vi "Feature_whole(SubVI)_TV.vi"(0 "Binary Image":T1) -> (4 "P":dbl, 5 "rgb Hull Image 2":T1(plugin-control), 6 "SA":dbl, 7 "bw Hull Image 2":T1(plugin-control), 8 "SFD":sgl, 9 "Hull area":dbl, 10 "SW":dbl, 12 "IFD":sgl, 13 "top":i32, 14 "最小外接矩面积":dbl, 15 "SH":dbl)   [LabVIEW 2015]
uses:
  <vilib>/vision/Image Controls.llb/IMAQ Image.ctl
  <vilib>/vision/NI_Vision_Development_Module.lvlib
  fractaldim.dll
  TotalContoursConvexHull.dll
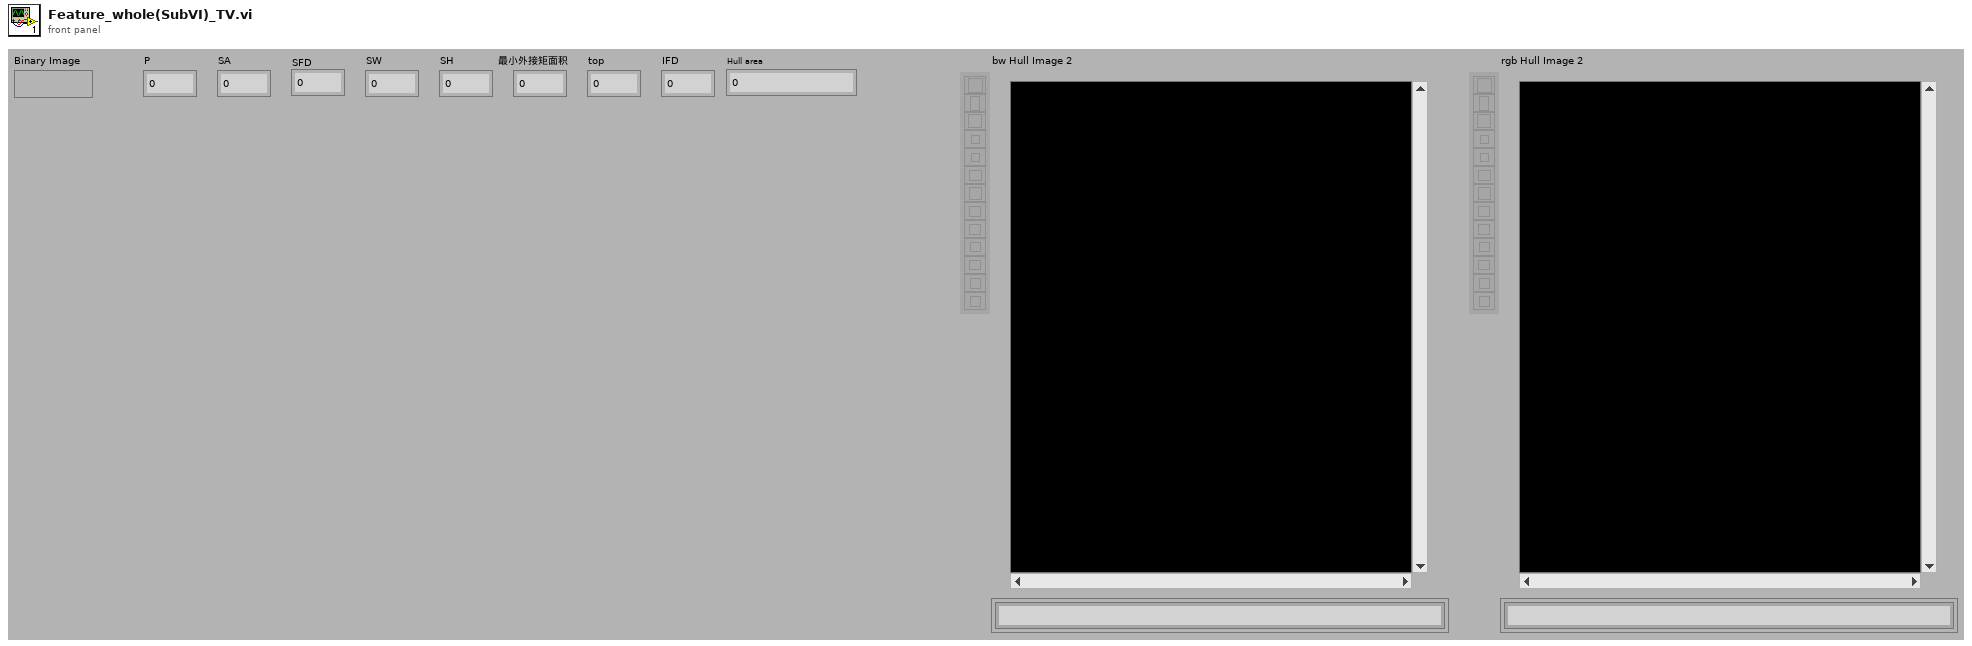
[diagram p1: front panel]
types:
  T1 = typedef "IMAQ Image.ctl" = refnum<image>
  T2 = typedef "Particle Parameters" = i32
  T3 = typedef "Image Type" = u32
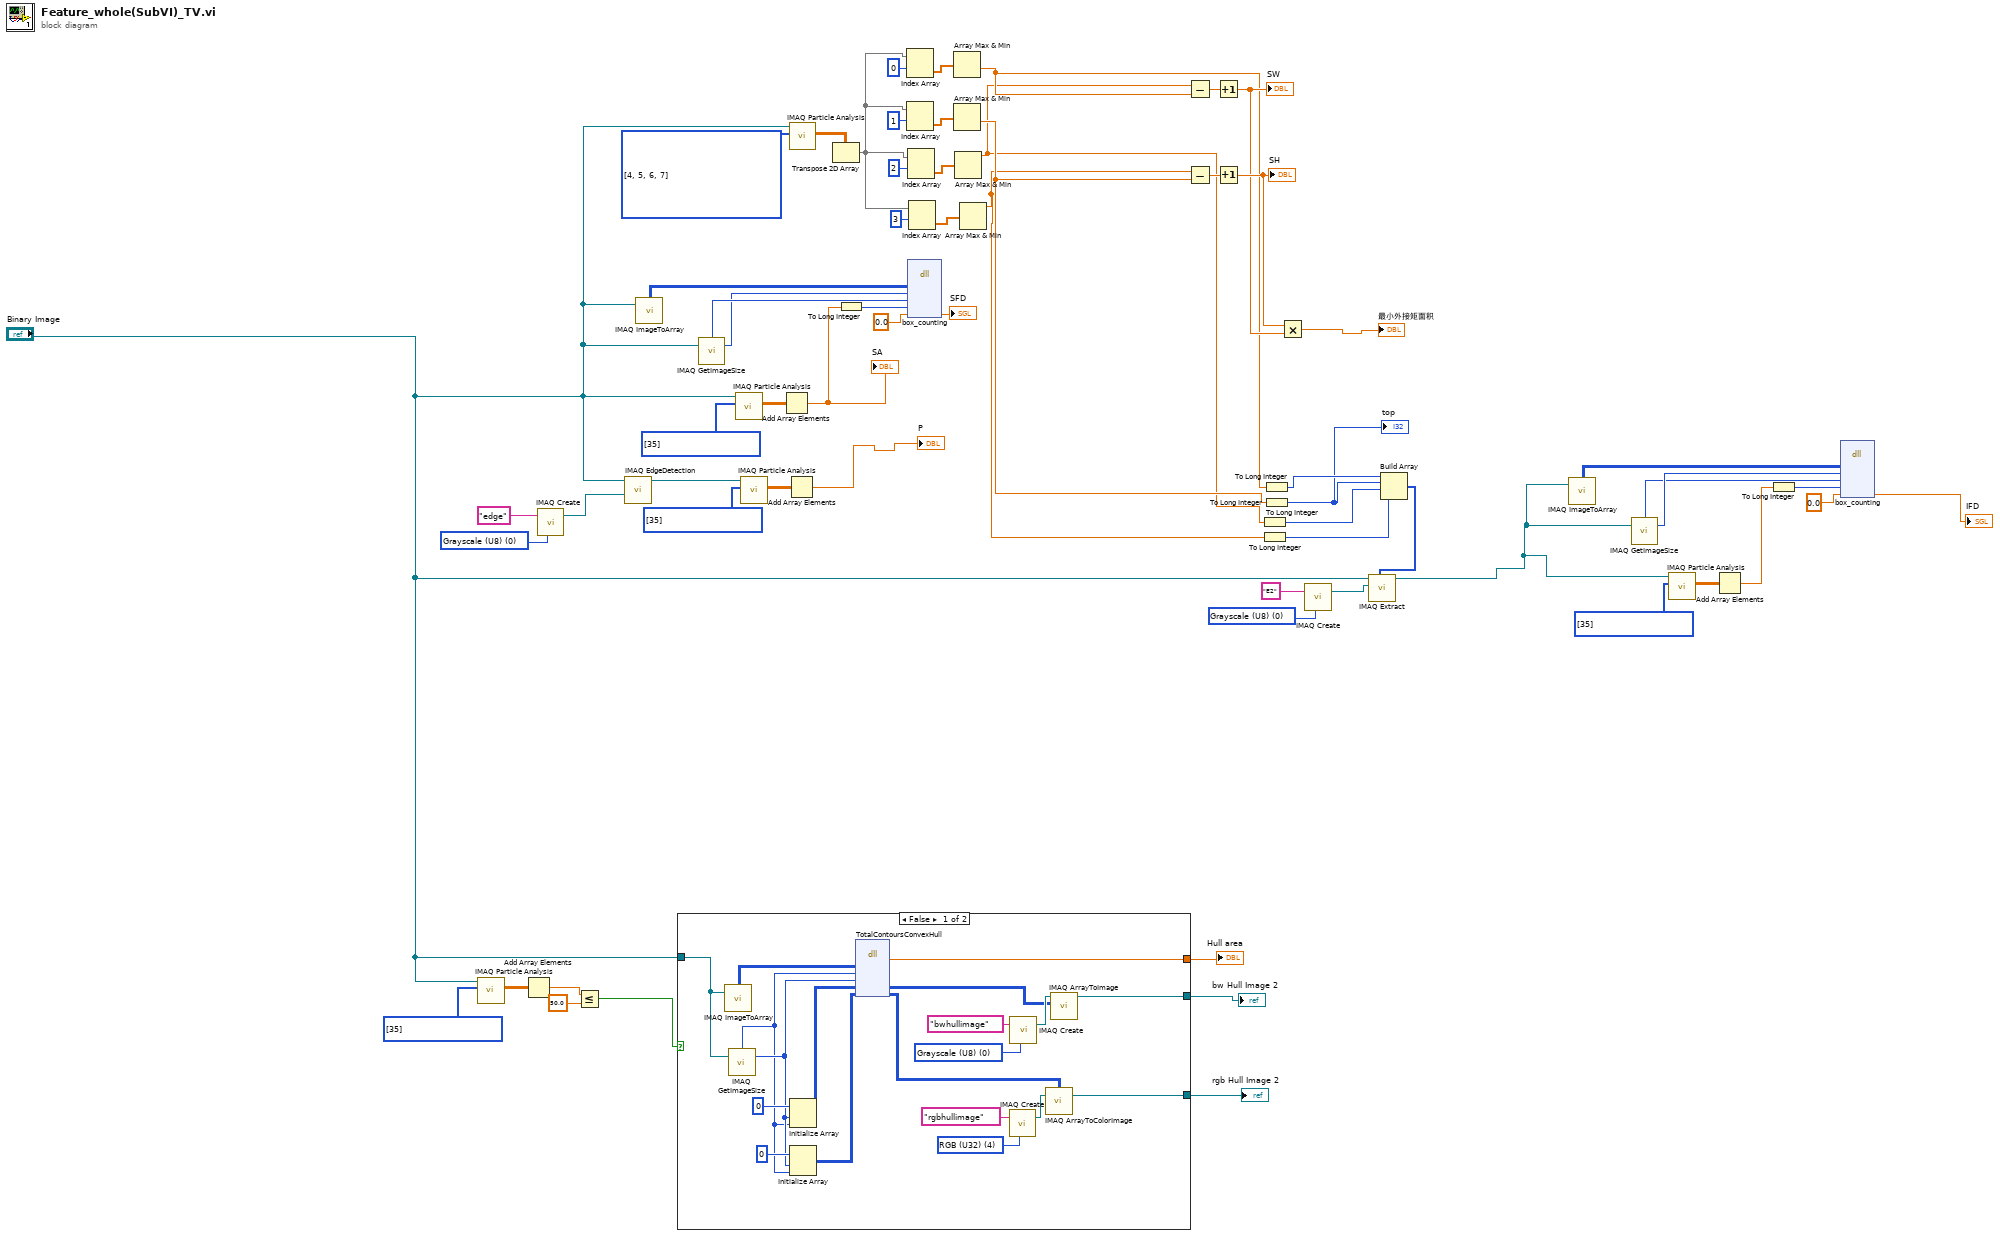
[diagram p0: block diagram]
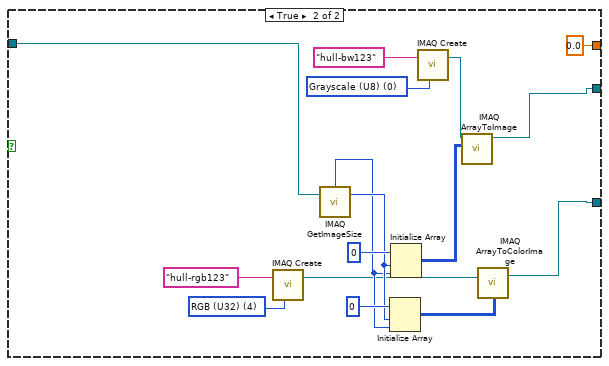
[diagram p2: hidden frame]
diagram:
  w7 = T2[] [35] items=["Center of Mass X", "Center of Mass Y", "First Pixel X", "First Pixel Y", "Bounding Rect Left", "Bounding Rect Top", "Bounding Rect Right", "Bounding Rect Bottom", "Max Feret Diameter Start X", "Max Feret Diameter Start Y", "Max Feret Diameter End X", "Max Feret Diameter End Y", "Max Horiz. Segment Length Left", "Max Horiz. Segment Length Right", "Max Horiz. Segment Length Row", "-", "Bounding Rect Width", "Bounding Rect Height", "Bounding Rect Diagonal", "Perimeter", "Convex Hull Perimeter", "Holes' Perimeter", "Max Feret Diameter", "Equivalent Ellipse Major Axis", "Equivalent Ellipse Minor Axis", "Equivalent Ellipse Minor Axis (Feret)", "Equivalent Rect Long Side", "Equivalent Rect Short Side", "Equivalent Rect Diagonal", "Equivalent Rect Short Side (Feret)", "Average Horiz. Segment Length", "Average Vert. Segment Length", "Hydraulic Radius", "Waddel Disk Diameter", "-", "Area", "Holes' Area", "Particle & Holes' Area", "Convex Hull Area", "Image Area", "-", "Number of Holes", "Number of Horiz. Segments", "Number of Vert. Segments", "-", "Orientation", "Max Feret Diameter Orientation", "-", "% Area/Image Area", "% Area/(Particle & Holes' Area)", "Ratio of Equivalent Ellipse Axes", "Ratio of Equivalent Rect Sides", "-", "Elongation Factor", "Compactness Factor", "Heywood Circularity Factor", "Type Factor", "-", "Sum X", "Sum Y", "Sum XX", "Sum XY", "Sum YY", "Sum XXX", "Sum XXY", "Sum XYY", "Sum YYY", "-", "Moment of Inertia XX", "Moment of Inertia XY", "Moment of Inertia YY", "Moment of Inertia XXX", "Moment of Inertia XXY", "Moment of Inertia XYY", "Moment of Inertia YYY", "Norm. Moment of Inertia XX", "Norm. Moment of Inertia XY", "Norm. Moment of Inertia YY", "Norm. Moment of Inertia XXX", "Norm. Moment of Inertia XXY", "Norm. Moment of Inertia XYY", "Norm. Moment of Inertia YYY", "Hu Moment 1", "Hu Moment 2", "Hu Moment 3", "Hu Moment 4", "Hu Moment 5", "Hu Moment 6", "Hu Moment 7"] ("Pixel Measurements")
  w56 = T2[] [35] items=["Center of Mass X", "Center of Mass Y", "First Pixel X", "First Pixel Y", "Bounding Rect Left", "Bounding Rect Top", "Bounding Rect Right", "Bounding Rect Bottom", "Max Feret Diameter Start X", "Max Feret Diameter Start Y", "Max Feret Diameter End X", "Max Feret Diameter End Y", "Max Horiz. Segment Length Left", "Max Horiz. Segment Length Right", "Max Horiz. Segment Length Row", "-", "Bounding Rect Width", "Bounding Rect Height", "Bounding Rect Diagonal", "Perimeter", "Convex Hull Perimeter", "Holes' Perimeter", "Max Feret Diameter", "Equivalent Ellipse Major Axis", "Equivalent Ellipse Minor Axis", "Equivalent Ellipse Minor Axis (Feret)", "Equivalent Rect Long Side", "Equivalent Rect Short Side", "Equivalent Rect Diagonal", "Equivalent Rect Short Side (Feret)", "Average Horiz. Segment Length", "Average Vert. Segment Length", "Hydraulic Radius", "Waddel Disk Diameter", "-", "Area", "Holes' Area", "Particle & Holes' Area", "Convex Hull Area", "Image Area", "-", "Number of Holes", "Number of Horiz. Segments", "Number of Vert. Segments", "-", "Orientation", "Max Feret Diameter Orientation", "-", "% Area/Image Area", "% Area/(Particle & Holes' Area)", "Ratio of Equivalent Ellipse Axes", "Ratio of Equivalent Rect Sides", "-", "Elongation Factor", "Compactness Factor", "Heywood Circularity Factor", "Type Factor", "-", "Sum X", "Sum Y", "Sum XX", "Sum XY", "Sum YY", "Sum XXX", "Sum XXY", "Sum XYY", "Sum YYY", "-", "Moment of Inertia XX", "Moment of Inertia XY", "Moment of Inertia YY", "Moment of Inertia XXX", "Moment of Inertia XXY", "Moment of Inertia XYY", "Moment of Inertia YYY", "Norm. Moment of Inertia XX", "Norm. Moment of Inertia XY", "Norm. Moment of Inertia YY", "Norm. Moment of Inertia XXX", "Norm. Moment of Inertia XXY", "Norm. Moment of Inertia XYY", "Norm. Moment of Inertia YYY", "Hu Moment 1", "Hu Moment 2", "Hu Moment 3", "Hu Moment 4", "Hu Moment 5", "Hu Moment 6", "Hu Moment 7"] ("Pixel Measurements")
  w26 = T3 0 items=["Grayscale (U8)", "Grayscale (I16)", "Grayscale (SGL)", "Complex (CSG)", "RGB (U32)", "HSL (U32)", "RGB (U64)", "Grayscale (U16)"] ("Image Type")
  w41 = T2[] [4, 5, 6, 7] items=["Center of Mass X", "Center of Mass Y", "First Pixel X", "First Pixel Y", "Bounding Rect Left", "Bounding Rect Top", "Bounding Rect Right", "Bounding Rect Bottom", "Max Feret Diameter Start X", "Max Feret Diameter Start Y", "Max Feret Diameter End X", "Max Feret Diameter End Y", "Max Horiz. Segment Length Left", "Max Horiz. Segment Length Right", "Max Horiz. Segment Length Row", "-", "Bounding Rect Width", "Bounding Rect Height", "Bounding Rect Diagonal", "Perimeter", "Convex Hull Perimeter", "Holes' Perimeter", "Max Feret Diameter", "Equivalent Ellipse Major Axis", "Equivalent Ellipse Minor Axis", "Equivalent Ellipse Minor Axis (Feret)", "Equivalent Rect Long Side", "Equivalent Rect Short Side", "Equivalent Rect Diagonal", "Equivalent Rect Short Side (Feret)", "Average Horiz. Segment Length", "Average Vert. Segment Length", "Hydraulic Radius", "Waddel Disk Diameter", "-", "Area", "Holes' Area", "Particle & Holes' Area", "Convex Hull Area", "Image Area", "-", "Number of Holes", "Number of Horiz. Segments", "Number of Vert. Segments", "-", "Orientation", "Max Feret Diameter Orientation", "-", "% Area/Image Area", "% Area/(Particle & Holes' Area)", "Ratio of Equivalent Ellipse Axes", "Ratio of Equivalent Rect Sides", "-", "Elongation Factor", "Compactness Factor", "Heywood Circularity Factor", "Type Factor", "-", "Sum X", "Sum Y", "Sum XX", "Sum XY", "Sum YY", "Sum XXX", "Sum XXY", "Sum XYY", "Sum YYY", "-", "Moment of Inertia XX", "Moment of Inertia XY", "Moment of Inertia YY", "Moment of Inertia XXX", "Moment of Inertia XXY", "Moment of Inertia XYY", "Moment of Inertia YYY", "Norm. Moment of Inertia XX", "Norm. Moment of Inertia XY", "Norm. Moment of Inertia YY", "Norm. Moment of Inertia XXX", "Norm. Moment of Inertia XXY", "Norm. Moment of Inertia XYY", "Norm. Moment of Inertia YYY", "Hu Moment 1", "Hu Moment 2", "Hu Moment 3", "Hu Moment 4", "Hu Moment 5", "Hu Moment 6", "Hu Moment 7"] ("Pixel Measurements")
  w48 = T2[] [35] items=["Center of Mass X", "Center of Mass Y", "First Pixel X", "First Pixel Y", "Bounding Rect Left", "Bounding Rect Top", "Bounding Rect Right", "Bounding Rect Bottom", "Max Feret Diameter Start X", "Max Feret Diameter Start Y", "Max Feret Diameter End X", "Max Feret Diameter End Y", "Max Horiz. Segment Length Left", "Max Horiz. Segment Length Right", "Max Horiz. Segment Length Row", "-", "Bounding Rect Width", "Bounding Rect Height", "Bounding Rect Diagonal", "Perimeter", "Convex Hull Perimeter", "Holes' Perimeter", "Max Feret Diameter", "Equivalent Ellipse Major Axis", "Equivalent Ellipse Minor Axis", "Equivalent Ellipse Minor Axis (Feret)", "Equivalent Rect Long Side", "Equivalent Rect Short Side", "Equivalent Rect Diagonal", "Equivalent Rect Short Side (Feret)", "Average Horiz. Segment Length", "Average Vert. Segment Length", "Hydraulic Radius", "Waddel Disk Diameter", "-", "Area", "Holes' Area", "Particle & Holes' Area", "Convex Hull Area", "Image Area", "-", "Number of Holes", "Number of Horiz. Segments", "Number of Vert. Segments", "-", "Orientation", "Max Feret Diameter Orientation", "-", "% Area/Image Area", "% Area/(Particle & Holes' Area)", "Ratio of Equivalent Ellipse Axes", "Ratio of Equivalent Rect Sides", "-", "Elongation Factor", "Compactness Factor", "Heywood Circularity Factor", "Type Factor", "-", "Sum X", "Sum Y", "Sum XX", "Sum XY", "Sum YY", "Sum XXX", "Sum XXY", "Sum XYY", "Sum YYY", "-", "Moment of Inertia XX", "Moment of Inertia XY", "Moment of Inertia YY", "Moment of Inertia XXX", "Moment of Inertia XXY", "Moment of Inertia XYY", "Moment of Inertia YYY", "Norm. Moment of Inertia XX", "Norm. Moment of Inertia XY", "Norm. Moment of Inertia YY", "Norm. Moment of Inertia XXX", "Norm. Moment of Inertia XXY", "Norm. Moment of Inertia XYY", "Norm. Moment of Inertia YYY", "Hu Moment 1", "Hu Moment 2", "Hu Moment 3", "Hu Moment 4", "Hu Moment 5", "Hu Moment 6", "Hu Moment 7"] ("Pixel Measurements")
  w51 = T3 0 items=["Grayscale (U8)", "Grayscale (I16)", "Grayscale (SGL)", "Complex (CSG)", "RGB (U32)", "HSL (U32)", "RGB (U64)", "Grayscale (U16)"] ("Image Type")
  w54 = T2[] [35] items=["Center of Mass X", "Center of Mass Y", "First Pixel X", "First Pixel Y", "Bounding Rect Left", "Bounding Rect Top", "Bounding Rect Right", "Bounding Rect Bottom", "Max Feret Diameter Start X", "Max Feret Diameter Start Y", "Max Feret Diameter End X", "Max Feret Diameter End Y", "Max Horiz. Segment Length Left", "Max Horiz. Segment Length Right", "Max Horiz. Segment Length Row", "-", "Bounding Rect Width", "Bounding Rect Height", "Bounding Rect Diagonal", "Perimeter", "Convex Hull Perimeter", "Holes' Perimeter", "Max Feret Diameter", "Equivalent Ellipse Major Axis", "Equivalent Ellipse Minor Axis", "Equivalent Ellipse Minor Axis (Feret)", "Equivalent Rect Long Side", "Equivalent Rect Short Side", "Equivalent Rect Diagonal", "Equivalent Rect Short Side (Feret)", "Average Horiz. Segment Length", "Average Vert. Segment Length", "Hydraulic Radius", "Waddel Disk Diameter", "-", "Area", "Holes' Area", "Particle & Holes' Area", "Convex Hull Area", "Image Area", "-", "Number of Holes", "Number of Horiz. Segments", "Number of Vert. Segments", "-", "Orientation", "Max Feret Diameter Orientation", "-", "% Area/Image Area", "% Area/(Particle & Holes' Area)", "Ratio of Equivalent Ellipse Axes", "Ratio of Equivalent Rect Sides", "-", "Elongation Factor", "Compactness Factor", "Heywood Circularity Factor", "Type Factor", "-", "Sum X", "Sum Y", "Sum XX", "Sum XY", "Sum YY", "Sum XXX", "Sum XXY", "Sum XYY", "Sum YYY", "-", "Moment of Inertia XX", "Moment of Inertia XY", "Moment of Inertia YY", "Moment of Inertia XXX", "Moment of Inertia XXY", "Moment of Inertia XYY", "Moment of Inertia YYY", "Norm. Moment of Inertia XX", "Norm. Moment of Inertia XY", "Norm. Moment of Inertia YY", "Norm. Moment of Inertia XXX", "Norm. Moment of Inertia XXY", "Norm. Moment of Inertia XYY", "Norm. Moment of Inertia YYY", "Hu Moment 1", "Hu Moment 2", "Hu Moment 3", "Hu Moment 4", "Hu Moment 5", "Hu Moment 6", "Hu Moment 7"] ("Pixel Measurements")
  n1 = call "IMAQ Particle Analysis"("Pixel Measurements"=w56, "Image"="Binary Image") -> ("Particle Measurements (Pixels)"=w57:dbl[][])  [unwired: 3 in, 6 out]
  n2 = Add Array Elements(numeric array=w57) -> (sum=w59:dbl)
  n3 = call "IMAQ Create"("Image Name"="edge", "Image Type"=w51) -> ("New Image"=w50:T1)  [unwired: 2 in, 2 out]
  n4 = Less Or Equal?(x=w59, y=50.0) -> (x <= y?=w60:bool)
  n5 = call "IMAQ EdgeDetection"("Image Dst"=w50, "Image Src"="Binary Image") -> ("Image Dst Out"=w53:T1)  [unwired: 4 in, 5 out]
  n6 = call "IMAQ ImageToArray"("Image"="Binary Image") -> ("Image Pixels (U8)"=w46:u8[][])  [unwired: 2 in, 5 out]
  n7 = case shown="False" w60 {
    tunnel: "Binary Image" -> [w67 w96]
    tunnel: [w66 0.0 ("areaSum")] -> w4
    tunnel: [w65 w94] -> w61
    tunnel: [w64 w83] -> w62
    frame False {
      w70 = T3 4 items=["Grayscale (U8)", "Grayscale (I16)", "Grayscale (SGL)", "Complex (CSG)", "RGB (U32)", "HSL (U32)", "RGB (U64)", "Grayscale (U16)"] ("Image Type")
      w80 = T3 0 items=["Grayscale (U8)", "Grayscale (I16)", "Grayscale (SGL)", "Complex (CSG)", "RGB (U32)", "HSL (U32)", "RGB (U64)", "Grayscale (U16)"] ("Image Type")
      n8 = call "IMAQ ImageToArray"("Image"=w67) -> ("Image Pixels (U8)"=w82:u8[][])  [unwired: 2 in, 5 out]
      n9 = call "IMAQ GetImageSize"("Image"=w67) -> ("Y Resolution"=w73:i32, "X Resolution"=w72:i32)  [unwired: 1 in, 3 out]
      n10 = Initialize Array(u8 0 ("element"), w73, w72) -> (w78:u8[][])
      n11 = Initialize Array(u32 0 ("element"), w73, w72) -> (w74:u32[][])
      n12 = dll-call lib="PTH2Tabs CUsersPCDesktop油菜顶视top_featuresTotalContoursConvexHull.dll" fn="TotalContoursConvexHull"("src"=w82, "width"=w72, "height"=w73, "bwhullimage"=w78, "rgbhullimage"=w74) -> ("areaSum"=w66:dbl, "bwhullimage"=w76:u8[][], "rgbhullimage"=w69:u32[][])  [unwired: 6 in, 2 out]
      n13 = call "IMAQ Create"("Image Name"="rgbhullimage", "Image Type"=w70) -> ("New Image"=w68:T1)  [unwired: 2 in, 2 out]
      n14 = call "IMAQ Create"("Image Name"="bwhullimage", "Image Type"=w80) -> ("New Image"=w79:T1)  [unwired: 2 in, 2 out]
      n15 = call "IMAQ ArrayToColorImage"("Image Pixels (U32)"=w69, "Image"=w68) -> ("Image Out"=w64:T1)  [unwired: 2 in, 2 out]
      n16 = call "IMAQ ArrayToImage"("Image Pixels (U8)"=w76, "Image"=w79) -> ("Image Out"=w65:T1)  [unwired: 4 in, 5 out]
    }
    frame True {
      w85 = T3 4 items=["Grayscale (U8)", "Grayscale (I16)", "Grayscale (SGL)", "Complex (CSG)", "RGB (U32)", "HSL (U32)", "RGB (U64)", "Grayscale (U16)"] ("Image Type")
      w93 = T3 0 items=["Grayscale (U8)", "Grayscale (I16)", "Grayscale (SGL)", "Complex (CSG)", "RGB (U32)", "HSL (U32)", "RGB (U64)", "Grayscale (U16)"] ("Image Type")
      n17 = call "IMAQ Create"("Image Name"="hull-rgb123", "Image Type"=w85) -> ("New Image"=w84:T1)  [unwired: 2 in, 2 out]
      n18 = call "IMAQ GetImageSize"("Image"=w96) -> ("Y Resolution"=w89:i32, "X Resolution"=w88:i32)  [unwired: 1 in, 3 out]
      n19 = Initialize Array(u32 0 ("element"), w89, w88) -> (w87:u32[][])
      n20 = Initialize Array(u8 0 ("element"), w89, w88) -> (w95:u8[][])
      n21 = call "IMAQ Create"("Image Name"="hull-bw123", "Image Type"=w93) -> ("New Image"=w91:T1)  [unwired: 2 in, 2 out]
      n22 = call "IMAQ ArrayToImage"("Image Pixels (U8)"=w95, "Image"=w91) -> ("Image Out"=w94:T1)  [unwired: 4 in, 5 out]
      n23 = call "IMAQ ArrayToColorImage"("Image Pixels (U32)"=w87, "Image"=w84) -> ("Image Out"=w83:T1)  [unwired: 2 in, 2 out]
    }
  }
  "Hull area" <- w4
  "bw Hull Image 2" <- w61
  "rgb Hull Image 2" <- w62
  n24 = call "IMAQ GetImageSize"("Image"="Binary Image") -> ("Y Resolution"=w42:i32, "X Resolution"=w43:i32)  [unwired: 1 in, 3 out]
  n25 = call "IMAQ Particle Analysis"("Pixel Measurements"=w48, "Image"="Binary Image") -> ("Particle Measurements (Pixels)"=w49:dbl[][])  [unwired: 3 in, 6 out]
  n26 = call "IMAQ Particle Analysis"("Pixel Measurements"=w54, "Image"=w53) -> ("Particle Measurements (Pixels)"=w55:dbl[][])  [unwired: 3 in, 6 out]
  n27 = Add Array Elements(numeric array=w49) -> (sum=w3:dbl)
  "SA" <- w3
  n28 = Add Array Elements(numeric array=w55) -> (sum=→"P":dbl)
  n29 = call "IMAQ Particle Analysis"("Pixel Measurements"=w41, "Image"="Binary Image") -> ("Particle Measurements (Pixels)"=w40:dbl[][])  [unwired: 3 in, 6 out]
  n30 = Transpose 2D Array(2D array=w40) -> (transposed array=w31:dbl[][])
  n31 = To Long Integer(number=w3) -> (32bit integer=w45:i32)
  n32 = Index Array(array=w31, index (row)=0) -> (element=w33:dbl[])  [unwired: 1 in]
  n33 = Index Array(array=w31, index (row)=1) -> (element=w34:dbl[])  [unwired: 1 in]
  n34 = Index Array(array=w31, index (row)=2) -> (element=w38:dbl[])  [unwired: 1 in]
  n35 = dll-call lib="PTH2Gabs CUsersPCDesktop油菜顶视top_featuresfractaldim.dll" fn="box_counting"("bw"=w46, "row"=w42, "col"=w43, "area"=w45, "FD"=sgl 0.0) -> ("FD"=→"SFD":sgl)  [unwired: 7 in, 3 out]
  n36 = Index Array(array=w31, index (row)=3) -> (element=w37:dbl[])  [unwired: 1 in]
  n37 = Array Max & Min(array=w33) -> (min value=w23:dbl)  [unwired: 3 out]
  n38 = Array Max & Min(array=w34) -> (min value=w21:dbl)  [unwired: 3 out]
  n39 = Array Max & Min(array=w38) -> (max value=w19:dbl)  [unwired: 3 out]
  n40 = Array Max & Min(array=w37) -> (max value=w17:dbl)  [unwired: 3 out]
  n41 = Subtract(x=w19, y=w23) -> (x-y=w30:dbl)
  n42 = Subtract(x=w17, y=w21) -> (x-y=w29:dbl)
  n43 = Increment(x=w30) -> (x+1=w27:dbl)
  "SW" <- w27
  n44 = Increment(x=w29) -> (x+1=w28:dbl)
  "SH" <- w28
  n45 = To Long Integer(number=w19) -> (32bit integer=w18:i32)
  n46 = To Long Integer(number=w17) -> (32bit integer=w16:i32)
  n47 = To Long Integer(number=w23) -> (32bit integer=w22:i32)
  n48 = To Long Integer(number=w21) -> (32bit integer=w20:i32)
  "top" <- w20
  n49 = Multiply(x=w28, y=w27) -> (x*y=→"最小外接矩面积":dbl)
  n50 = call "IMAQ Create"("Image Name"="E2", "Image Type"=w26) -> ("New Image"=w24:T1)  [unwired: 2 in, 2 out]
  n51 = Build Array(w22, w20, w18, w16) -> (w15:i32[])
  n52 = call "IMAQ Extract"("Optional Rectangle"=w15, "Image Dst"=w24, "Image Src"="Binary Image") -> ("Image Dst Out"=w14:T1)  [unwired: 3 in, 5 out]
  n53 = call "IMAQ ImageToArray"("Image"=w14) -> ("Image Pixels (U8)"=w9:u8[][])  [unwired: 2 in, 5 out]
  n54 = call "IMAQ GetImageSize"("Image"=w14) -> ("Y Resolution"=w12:i32, "X Resolution"=w11:i32)  [unwired: 1 in, 3 out]
  n55 = call "IMAQ Particle Analysis"("Pixel Measurements"=w7, "Image"=w14) -> ("Particle Measurements (Pixels)"=w6:dbl[][])  [unwired: 3 in, 6 out]
  n56 = Add Array Elements(numeric array=w6) -> (sum=w13:dbl)
  n57 = To Long Integer(number=w13) -> (32bit integer=w10:i32)
  n58 = dll-call lib="PTH2Gabs CUsersPCDesktop油菜顶视top_featuresfractaldim.dll" fn="box_counting"("bw"=w9, "row"=w12, "col"=w11, "area"=w10, "FD"=sgl 0.0) -> ("FD"=→"IFD":sgl)  [unwired: 7 in, 3 out]
